vi "Update_random_B.vi"(8 "error in (no error)":errorcluster, 10 "Random":u64, 11 "B_Actor in":refnum<class "B_Actor.lvclass">) -> (0 "error out":errorcluster, 3 "B_Actor out":refnum<class "B_Actor.lvclass">)   [LabVIEW 2025, in "B_Actor.lvlib" / "B_Actor.lvclass"]
uses:
  B_Actor.lvclass
  B_Actor.lvclass/B_Actor.ctl
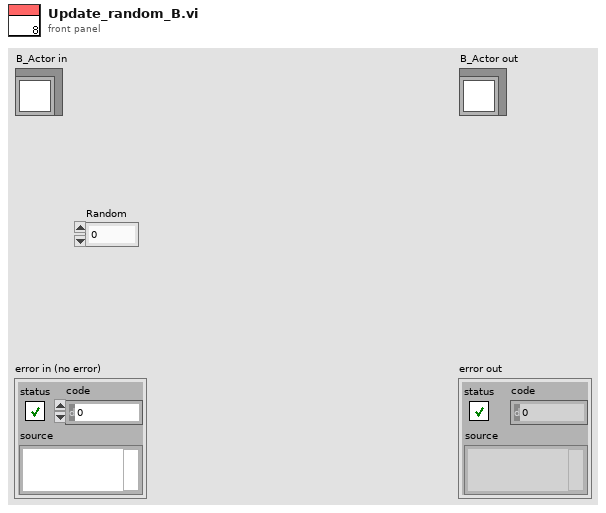
[diagram p1: front panel]
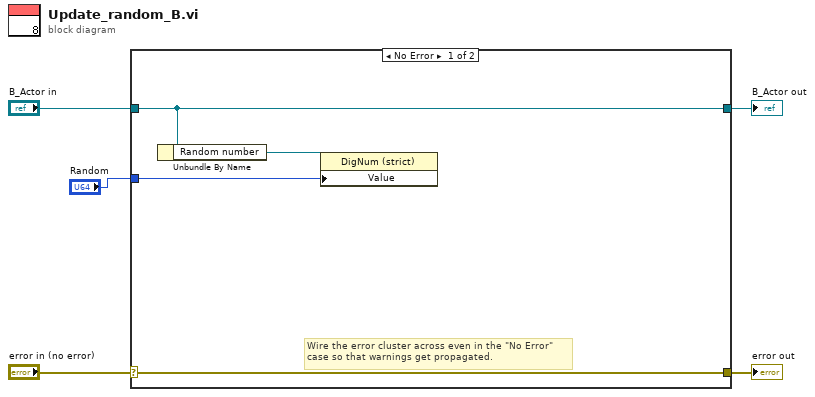
[diagram p0: block diagram]
diagram:
  n1 = case shown="No Error" "error in (no error)" {
    selector: "error in (no error)" -> [w9 w11]
    tunnel: [w9 w11] -> w4
    tunnel: [w8 w10] -> w2
    tunnel: "B_Actor in" -> [w8 w10]
    tunnel: "Random" -> [w6 _]
    frame No Error {
      # "Wire the error cluster across even in the \"No Error\"\ncase so that warnings get propagated."
      n2 = Unbundle By Name(w8) -> ("Random number"=w7:refnum<vi>)
      n3 = property class="DigNum (strict)"(reference=w7, "Value"=w6) -> ()  [unwired: 1 in, 2 out]
    }
    frame Error {
    }
  }
  "error out" <- w4
  "B_Actor out" <- w2
